vi "SimplePythonTest.vi"() -> ()   [LabVIEW 2019]
uses:
  <userlib>/MicroPython/VIs/SSH/PythonVersion.vi
panel:
  out "para read":string
  out "return value":string
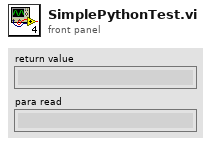
[diagram p1: front panel]
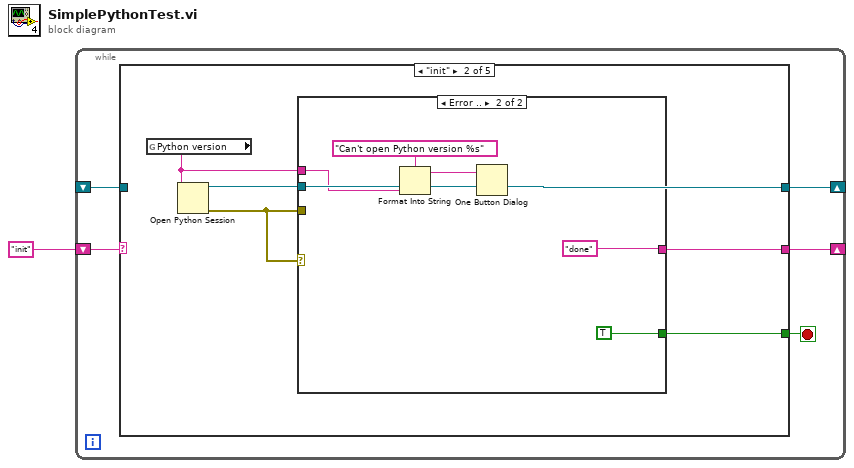
[diagram p0: block diagram]
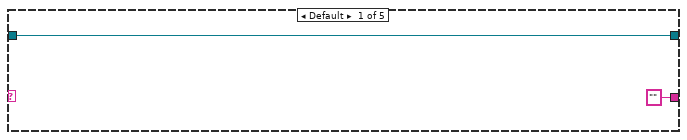
[diagram p2: hidden frame]
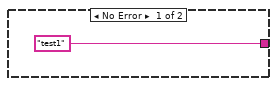
[diagram p3: hidden frame]
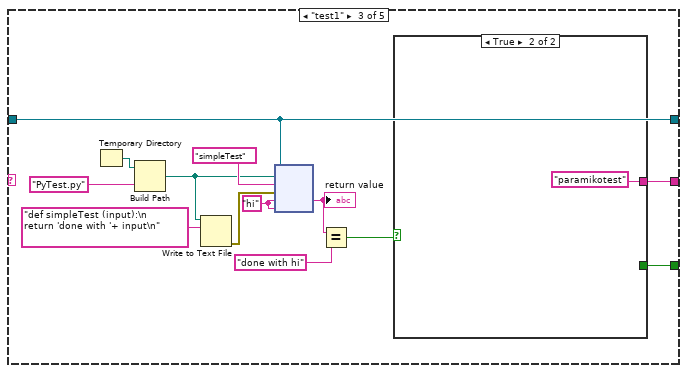
[diagram p4: hidden frame]
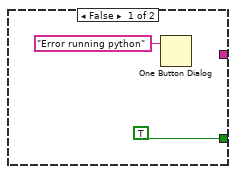
[diagram p5: hidden frame]
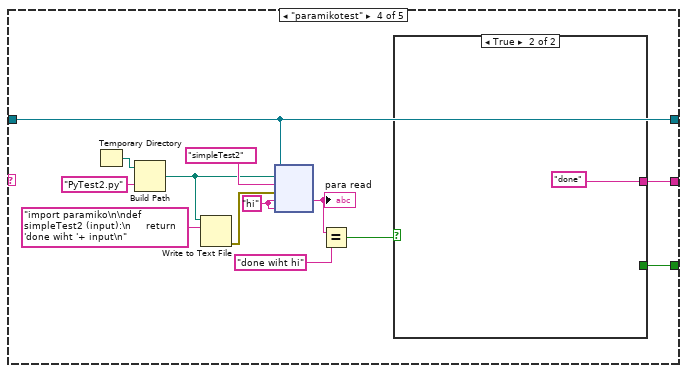
[diagram p6: hidden frame]
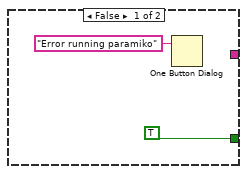
[diagram p7: hidden frame]
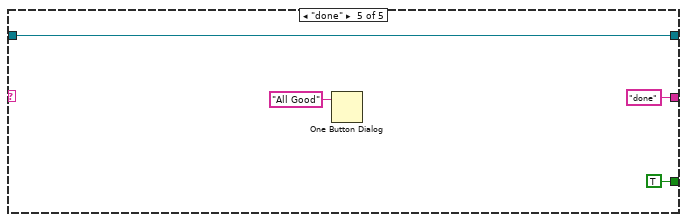
[diagram p8: hidden frame]
diagram:
  n1 = while {
    shift-right: [w4] -> _
    shift-left: "init" ("name or relative path") -> [w5]
    shift-right: [w3] -> _
    shift-left: _ -> [w2]
    stop <- w6 stop-if-true
    n2 = case shown="\"init\"" w5 {
      tunnel: [_ w12 w20 w36 TRUE] -> w6
      tunnel: ["" ("return value") w11 w22 w38 "done" ("return value")] -> w4
      tunnel: [w8 w10 w23 w39 w55] -> w3
      tunnel: w2 -> [w8 _ w23 w39 w55]
      frame Default {
      }
      frame "init" {
        n3 = global read "PythonVersion.vi" "Python version"() -> (w9:string)
        n4 = Open Python Session(python version=w9) -> (session out=w10:refnum<k35>, error out=w13:errorcluster)  [unwired: 2 in]
        n5 = case shown="Error .." w13 {
          tunnel: w10 -> [_ _]
          tunnel: w13 -> [_ _]
          tunnel: [_ TRUE] -> w12
          tunnel: ["test1" ("name or relative path") "done" ("name or relative path")] -> w11
          tunnel: w9 -> [_ w17]
          frame No Error {
          }
          frame Error {
            n6 = Format Into String(format string="Can't open Python version %s" ("message"), w17) -> (resulting string=w15:string)  [unwired: 2 in, 1 out]
            n7 = One Button Dialog(message=w15) -> ()  [unwired: 1 in, 1 out]
          }
        }
      }
      frame "test1" {
        w29 = "hi" ("function name")
        n8 = Temporary Directory() -> (w28:path)
        n9 = Build Path(base path=w28, name or relative path="PyTest.py") -> (appended path=w26:path)
        n10 = Write to Text File(file (use dialog)=w26, text="def simpleTest (input):\n     return 'done with '+ input\n" ("name or relative path")) -> (error out=w30:errorcluster)  [unwired: 2 in, 2 out]
        n11 = node(w23, w26, "simpleTest" ("function name"), w30, w29, w29) -> (w24:string)  [unwired: 1 in, 4 out]
        "return value" <- w24
        n12 = Equal?(x=w24, y="done with hi" ("return value")) -> (x = y?=w21:bool)
        n13 = case shown="True" w21 {
          tunnel: [_ "paramikotest" ("return value")] -> w22
          tunnel: [TRUE _] -> w20
          frame False {
            n14 = One Button Dialog(message="Error running python") -> ()  [unwired: 1 in, 1 out]
          }
          frame True {
          }
        }
      }
      frame "paramikotest" {
        w45 = "hi" ("function name")
        n15 = Temporary Directory() -> (w44:path)
        n16 = Build Path(base path=w44, name or relative path="PyTest2.py") -> (appended path=w42:path)
        n17 = Write to Text File(file (use dialog)=w42, text="import paramiko\n\ndef simpleTest2 (input):\n     return 'done wiht '+ input\n" ("name or relative path")) -> (error out=w46:errorcluster)  [unwired: 2 in, 2 out]
        n18 = node(w39, w42, "simpleTest2" ("function name"), w46, w45, w45) -> (w40:string)  [unwired: 1 in, 4 out]
        "para read" <- w40
        n19 = Equal?(x=w40, y="done wiht hi" ("return value")) -> (x = y?=w37:bool)
        n20 = case shown="True" w37 {
          tunnel: [_ "done" ("return value")] -> w38
          tunnel: [TRUE _] -> w36
          frame False {
            n21 = One Button Dialog(message="Error running paramiko") -> ()  [unwired: 1 in, 1 out]
          }
          frame True {
          }
        }
      }
      frame "done" {
        n22 = One Button Dialog(message="All Good") -> ()  [unwired: 1 in, 1 out]
      }
    }
  }
